vi "Manipulating Arrays.vi"() -> ()   [LabVIEW 2020]
uses:
  <vilib>/DAQmx/read.llb/DAQmx Read (Analog 1D DBL 1Chan NSamp).vi
  <vilib>/DAQmx/create/channels.llb/DAQmx Create Channel (AI-Acceleration-Accelerometer).vi
  <vilib>/DAQmx/configure/timing.llb/DAQmx Timing (Sample Clock).vi
  <vilib>/DAQmx/miscellaneous.llb/DAQmx Fill In Error Info.vi
panel:
  out "Delete From Array":dbl[](array[numeric])
  out "Insert Into Array Result":dbl[](array[numeric])
  out "Replace Array Subset Result":dbl[](array[numeric])
  out "Single Element":dbl
  out "Array Length":i32
  out "Acceleration Data - Graph":dbl[](graph)
  out "Acceleration Data - Array":dbl[](array[numeric])
  # "(3rd Element)"
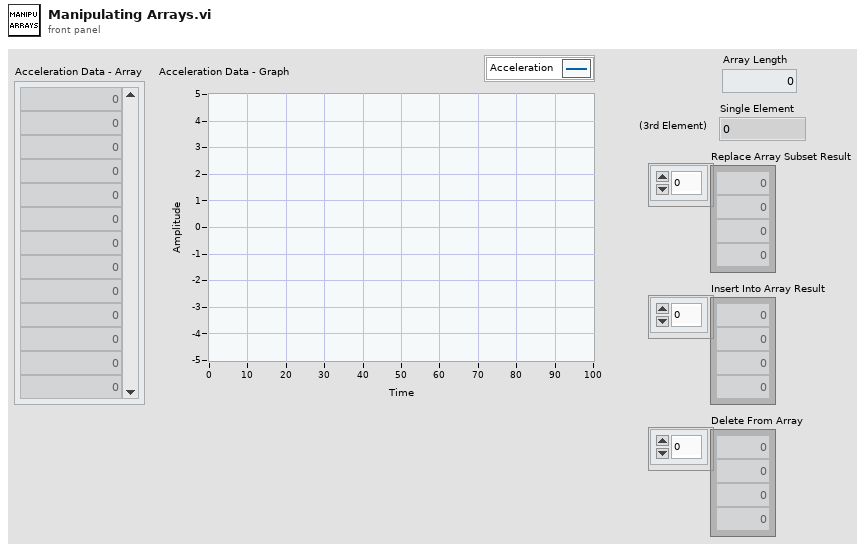
[diagram p1: front panel]
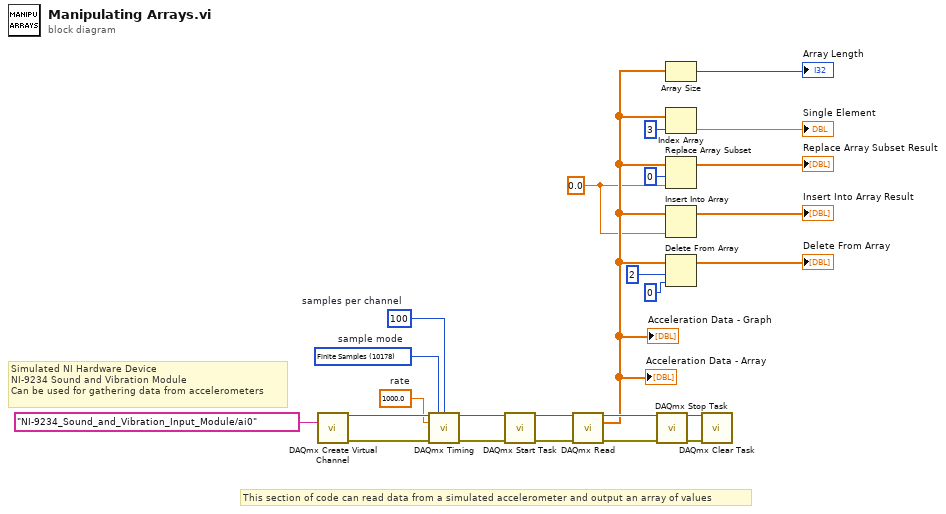
[diagram p0: block diagram]
diagram:
  w3 = 0.0 ("new element/subarray")
  w12 = 1000.0  # rate
  w13 = 100  # samples per channel
  w14 = 10178 items=["Finite Samples"=10178, "Continuous Samples"=10123, "Hardware Timed Single Point"=12522]  # sample mode
  # "This section of code can read data from a simulated accelerometer and output an array of values"
  # "Simulated NI Hardware Device\nNI-9234 Sound and Vibration Module\nCan be used for gathering data from accelerometers"
  n1 = call-poly <vilib>:"DAQmx Create Virtual Channel.vi"("physical channels"=tag "NI-9234_Sound_and_Vibration_Input_Module/ai0") -> ("task out"=w18:refnum<k21>, "error out"=w17:errorcluster)  [unwired: 13 in]
  n2 = call-poly <vilib>:"DAQmx Timing.vi"("task/channels in"=w18, "sample mode"=w14, "samples per channel"=w13, "rate"=w12, "error in"=w17) -> ("task out"=w16:refnum<k21>, "error out"=w15:errorcluster)  [unwired: 9 in]
  n3 = call <vilib>:"DAQmx Start Task.vi"("task/channels in"=w16, "error in"=w15) -> ("task out"=w24:refnum<k21>, "error out"=w25:errorcluster)  [unwired: 12 in]
  n4 = call-poly <vilib>:"DAQmx Read.vi"("task/channels in"=w24, "error in"=w25) -> ("task out"=w22:refnum<k21>, "data"=w11:dbl[], "error out"=w21:errorcluster)  [unwired: 11 in]
  "Acceleration Data - Array" <- w11
  "Acceleration Data - Graph" <- w11
  n5 = call <vilib>:"DAQmx Stop Task.vi"("task/channels in"=w22, "error in"=w21) -> ("task out"=w23:refnum<k21>, "error out"=w20:errorcluster)  [unwired: 12 in]
  n6 = Array Size(array=w11) -> (size(s)=→"Array Length":i32)
  n7 = Index Array "Index Array"(array=w11, index=3) -> (element=→"Single Element":dbl)
  n8 = Replace Array Subset "Replace Array Subset"(array=w11, new element=w3, index=0) -> (→"Replace Array Subset Result":dbl[])
  n9 = Insert Into Array "Insert Into Array"(array=w11, new element=w3) -> (→"Insert Into Array Result":dbl[])  [unwired: 1 in]
  n10 = Delete From Array "Delete From Array"(array=w11, length=2, index=0) -> (array with subset deleted=→"Delete From Array":dbl[])  [unwired: 1 out]
  n11 = call <vilib>:"DAQmx Clear Task.vi"("task in"=w23, "error in"=w20) -> ()  [unwired: 13 in, 1 out]
